vi "timestamp.vi"() -> ()   [LabVIEW 2020]
panel:
  out "seconds":dbl=3710947362.4402113
  in  "timestamp":timestamp=timestamp(3710947362.4402113 s since 1904-01-01) format="%<%Y-%m-%dT%H:%M:%S>T"
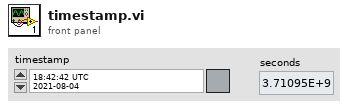
[diagram p1: front panel]
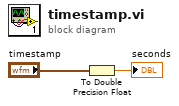
[diagram p0: block diagram]
diagram:
  n1 = To Double Precision Float(number="timestamp") -> (double precision float=→"seconds":dbl)
